vi "get_daq_resources.vi"(8 "error in (no error)":errorcluster) -> (0 "error out":errorcluster, 2 "Resources out":refnum<k20>[](array[refnum]), 3 "Refnum out":refnum<k21>)   [LabVIEW 2015]
uses:
  <vilib>/nisyscfg/nisyscfg.lvlib
  <resource>/objmgr/nisysapi.rc
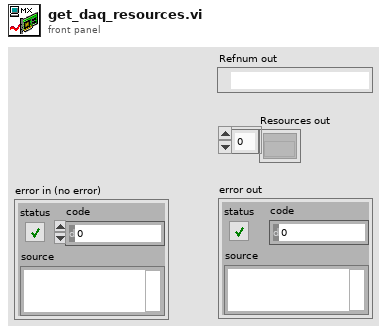
[diagram p1: front panel]
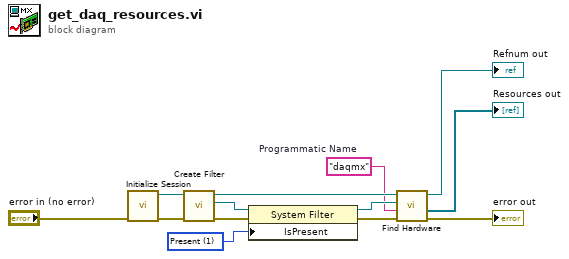
[diagram p0: block diagram]
diagram:
  w5 = 1 items=["Unknown"=-1, "Not Present"=0, "Present"=1] ("Is Present")
  w1 = "daqmx"  # Programmatic Name
  n1 = call <vilib>:"Initialize Session.vi"("error in (no error)"="error in (no error)") -> ("error out"=w3:errorcluster, "Session out"=w4:refnum<k21>)  [unwired: 9 in]
  n2 = call <vilib>:"Create Filter.vi"("error in (no error)"=w3, "Session in"=w4) -> ("error out"=w8:errorcluster, "Filter out"=w9:refnum<k20>, "Session out"=w2:refnum<k21>)  [unwired: 7 in]
  n3 = property class="System Filter"(reference=w9, error in=w8, "IsPresent"=w5) -> (reference out=w6:refnum<k20>, error out=w7:errorcluster)
  n4 = call <vilib>:"Find Hardware.vi"("error in (no error)"=w7, "Experts"=w1, "Filter in"=w6, "Session in"=w2) -> ("error out"=→"error out":errorcluster, "Resources out"=→"Resources out":refnum<k20>[], "Session out"=→"Refnum out":refnum<k21>)  [unwired: 4 in, 1 out]
